vi "运维调试_CODCr.vi"() -> ()   [LabVIEW 2016, in "CODCr库.lvlib"]
uses:
  <vilib>/Utility/miscctls.llb/LVPointTypeDef.ctl
  <vilib>/ptbypt/NI_PtbyPt.lvlib
  <vilib>/Utility/config.llb/NI_LVConfig.lvlib
panel:
  out "数据时间":timestamp format="%<%Y/%m/%d %H:%M:%S>T"
  in  "质控参数":bool
  in  "仪器参数":bool
  in  "MB通信方式选择":enum16{"串口", "TCP"}(ring)
  in  "释放串口":bool
  in  "打开串口":bool
  in  "加标回收测试":bool
  in  "平行样测试":bool
  in  "定时启动":bool
  out "COM口":string
  in  "空白测试":bool
  in  "隐藏按钮":bool
  in  "写入消解温度时长":bool
  in  "保存KB值":bool
  in  "标样核查":bool
  out "启动时间":timestamp format="%<%Y/%m/%d %H:%M:%S>T"
  out "主循环次数":i32
  out "status":bool
  out "启动测量模式":T1(ring)
  out "曲线截距B":sgl format="%#_10g"
  out "曲线斜率K":sgl format="%#_10g"
  out "量程上限":sgl
  out "量程下限":sgl
  out "消解时长":u16
  out "消解温度":u16
  out "测量精度":u16
  out "测量结果":sgl
  out "标样参考值":sgl
  out "量程":u16
  out "工作状态":T1(ring)
  out "仪器时间":timestamp format="%<%X\n%x>T"
  out "关键参数区":T2
  out "状态告警区":T3 {"告警代码" items=["无告警", "缺试剂告警", "缺水样告警", "缺蒸馏水告警", "缺标液告警", "仪表漏液告警", "标定异常告警", "超量程告警", "加热异常", "低试剂预警", "超上限告警", "超下限告警", "仪表内部其他异常", "滴定异常告警", "电极异常告警", "量程切换告警", "参数设置告警", "PH电极电位异常", "电导率电极异常", "浊度光度异常", "溶解氧电极异常", "溶解氧光强异常", "温度异常告警", "PH异常告警", "溶解氧异常告警", "电导率异常告警", "浊度异常告警", "叶绿素异常告警", "藻密度异常告警", "蓝绿藻异常告警", "ORP异常告警", "氨氮异常告警", "清洁刷异常告警", "SD卡异常告警", "蓝牙异常告警", "Wifi异常告警", "流程异常告警"]; "故障代码" items=["无故障", "电机故障", "温度故障", "通讯故障", "滴定故障"]}
  out "测量数据区":T4 {"单位" items=["ug/L", "mg/L", "ppm", "mg/m3", "cm", "ppb", "ug/m3", "%", "nmol/mol", "umol/mol", "MPN/L", "MPN/100ml", "ng/m3", "NTU", "无量纲", "ms/cm", "us/cm", "℃", "mV", "万个/L"]}
  out "系统时间":timestamp format="%<%Y/%m/%d %H:%M:%S>T"
  in  "停止":bool
  in  "校时":bool
  in  "标样校准":bool
  in  "空白校准":bool
  in  "零点核查":bool
  in  "跨度核查":bool
  in  "水样测试":bool
  in  "返回":bool
  in  "设置":bool
  # "mg/L"
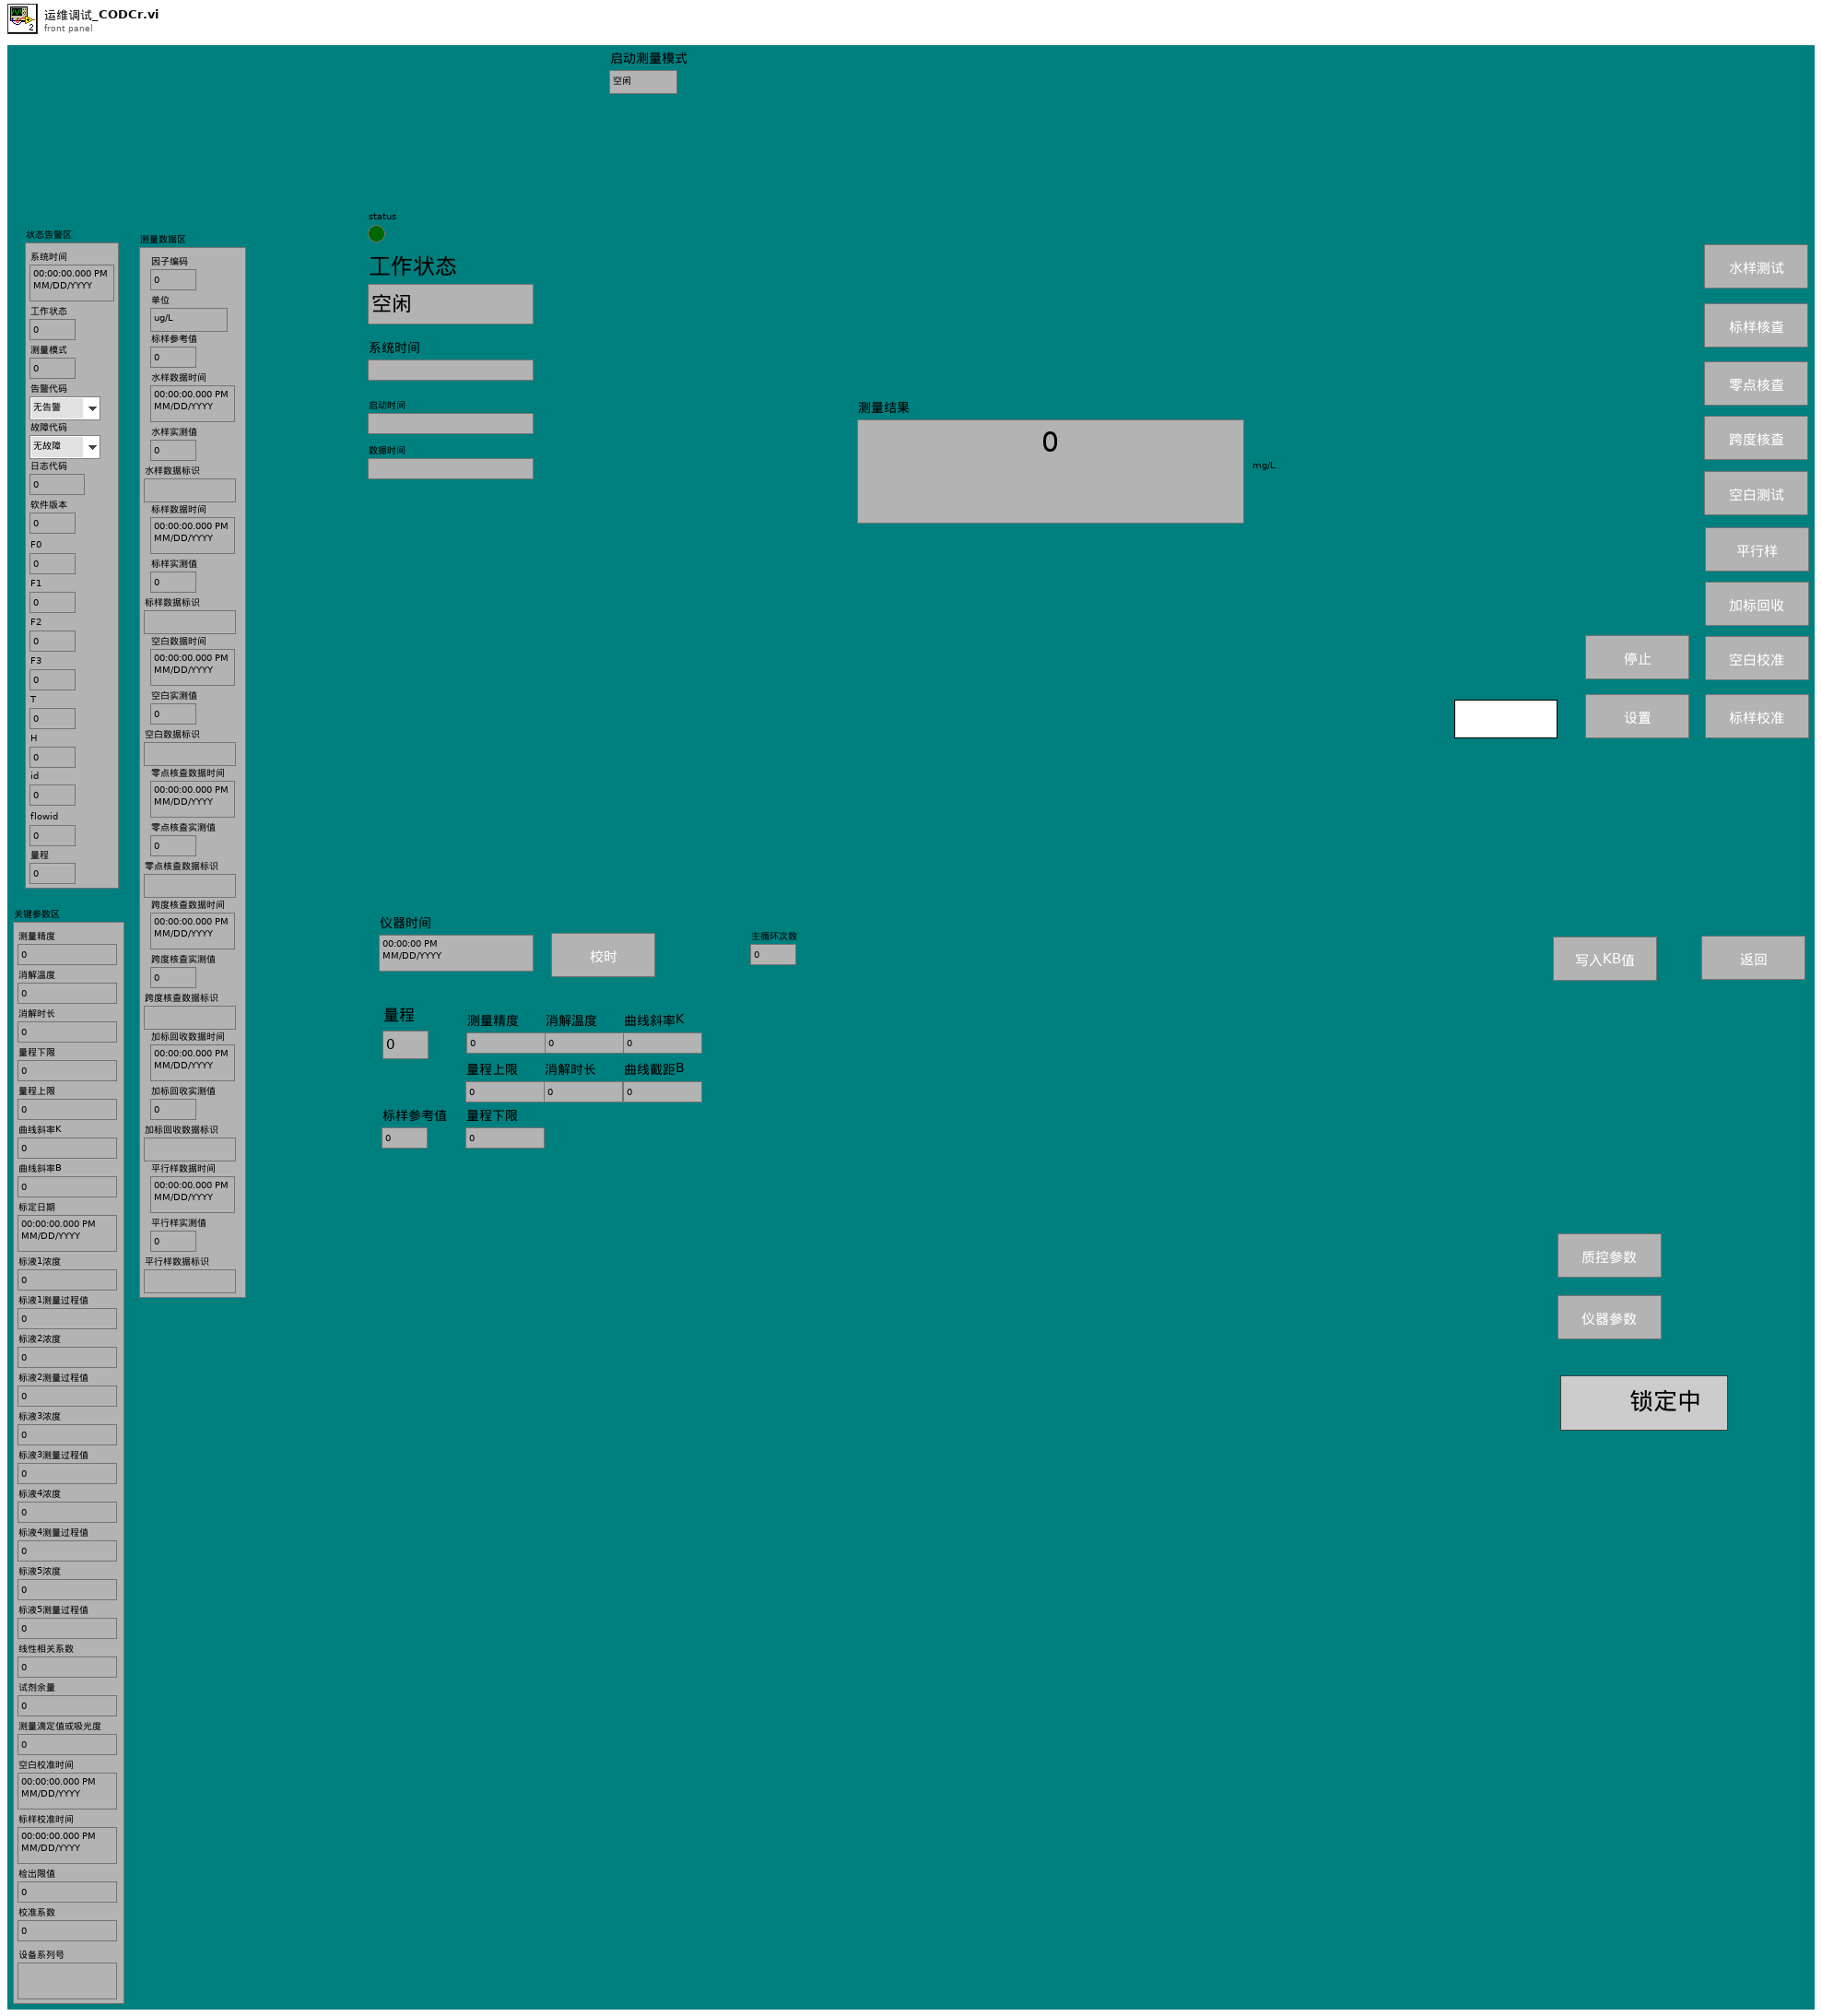
[diagram p1: front panel]
types:
  T1 = enum16{"空闲", "水样测试", "标样核查", "零点核查", "跨度核查", "空白测试", "平行样测试", "加标回收", "空白校准", "标样校准", "初始化（清洗）"}
  T2 = cluster{"测量精度":u16, "消解温度":u16, "消解时长":u16, "量程下限":sgl, "量程上限":sgl, "曲线斜率K":sgl, "曲线斜率B":sgl, "标定日期":timestamp, "标液1浓度":sgl, "标液1测量过程值":sgl, "标液2浓度":sgl, "标液2测量过程值":sgl, "标液3浓度":sgl, "标液3测量过程值":sgl, "标液4浓度":sgl, "标液4测量过程值":sgl, "标液5浓度":sgl, "标液5测量过程值":sgl, "线性相关系数":sgl, "试剂余量":u32, "测量滴定值或吸光度":sgl, "空白校准时间":timestamp, "标样校准时间":timestamp, "检出限值":sgl, "校准系数":sgl, "设备系列号":string}
  T3 = cluster{"系统时间":timestamp, "工作状态":u16, "测量模式":u16, "告警代码":u16, "故障代码":u16, "日志代码":u16, "软件版本":u16, "F0":sgl, "F1":sgl, "F2":sgl, "F3":sgl, "T":sgl, "H":sgl, "id":u16, "flowid":u16, "量程":u16}
  T4 = cluster{"因子编码":u32, "单位":u16, "标样参考值":sgl, "水样数据时间":timestamp, "水样实测值":sgl, "水样数据标识":string, "标样数据时间":timestamp, "标样实测值":sgl, "标样数据标识":string, "空白数据时间":timestamp, "空白实测值":sgl, "空白数据标识":string, "零点核查数据时间":timestamp, "零点核查实测值":sgl, "零点核查数据标识":string, "跨度核查数据时间":timestamp, "跨度核查实测值":sgl, "跨度核查数据标识":string, "加标回收数据时间":timestamp, "加标回收实测值":sgl, "加标回收数据标识":string, "平行样数据时间":timestamp, "平行样实测值":sgl, "平行样数据标识":string}
  T5 = cluster{"命令":string, "测量模式":enum16{"水样测量", "标样核查", "零点核查", "跨度核查", "空白测试", "加标回收", "平行样", "校零", "校标"}, "CODCr量程切换":enum32{"H", "L", "AUTO"}}
  T6 = typedef "LVPointTypeDef.ctl" = cluster{"Horizontal":i16, "Vertical":i16}
  T7 = typedef "NI_LVConfig.lvlib/Config Data RefNum.ctl" = refnum<k1>
  T8 = enum8{"Enabled", "Disabled", "Disabled and Grayed Out"}
  T9 = cluster{"运行模式":enum16{"维护模式", "常规模式", "应急模式", "质控模式"}}
  T10 = cluster{"时间标识":timestamp, "监测值":sgl, "单位":u16, "数据标识":string, "因子编码":u32, "标样参考值":sgl, "F0":sgl, "F1":sgl, "F2":sgl, "F3":sgl, "温度":sgl, "湿度":sgl, "量程标识":string, "LastTime":timestamp}
  T11 = cluster{"时间标识":timestamp, "设备":string, "日志信息":string}
  T12 = cluster{"时间标识":timestamp, "参数":string, "日志信息":string, "流程参数":string}
  T13 = cluster{"时间标识":timestamp, "设备":string, "日志信息":string, "流程参数":string}
  T14 = enum16{"水样测量", "标样核查", "零点核查", "跨度核查", "空白测试", "加标回收", "平行样", "校零", "校标"}
  T15 = cluster{"控制命令":enum16{"启动测量", "标样核查", "零点核查", "跨度核查", "空白测试", "平行样测试", "加标回收", "空白校准", "标样校准", "初始化（清洗）", "停止测试", "仪器重启", "校时", "模式设置", "测量间隔设置"}, "周期设置类型":enum16{"定点启动", "间隔启动"}, "定时功能启用":bool, "定时间隔":dbl, "24H周期设置":bool[], "零点核查时间":u16, "跨度核查时间":u16, "质控频次":enum16{"关闭", "每天", "星期一", "星期二", "星期三", "星期四", "星期五", "星期六", "星期日"}}
  T16 = cluster{"测量量程":dbl, "测量精度":dbl, "测量间隔":dbl, "消解温度":dbl, "消解时长":dbl, "空白校准时间":timestamp, "曲线截距":dbl, "曲线斜率":dbl, "测量检出限":dbl, "测量信号值":dbl, "线性相关系数":dbl, "二次多项式系数":dbl, "标样校准时间":timestamp, "稀释倍数":dbl, "三项式系数":dbl, "空白标定系数":dbl, "量程系数":dbl, "F0/ORPA":dbl, "F1/ORPB":dbl, "F2/ORPK":dbl, "F3":dbl, "F4":dbl, "F5":dbl, "F6":dbl, "F7":dbl, "X0/滴定数":dbl, "量程":dbl}
  T17 = cluster{"控制命令":enum16{"启动测量", "标样核查", "零点核查", "跨度核查", "空白测试", "平行样测试", "加标回收", "空白校准", "标样校准", "初始化（清洗）", "停止测试", "仪器重启", "校时", "模式设置", "测量间隔设置"}, "周期设置类型":enum16{"定点启动", "间隔启动"}, "定时功能启用":bool, "定时间隔":dbl, "24H周期设置":bool[], "空白核查时间":u16, "跨度核查时间":u16, "质控频次":enum16{"关闭", "每天", "星期一", "星期二", "星期三", "星期四", "星期五", "星期六", "星期日"}}
  T18 = cluster{"确定":bool, "测量量程":dbl, "测量精度":dbl, "测量间隔":dbl, "消解温度":dbl, "消解时长":dbl, "空白校准时间":timestamp, "曲线截距":dbl, "曲线斜率":dbl, "测量检出限":dbl, "测量信号值":dbl, "线性相关系数":dbl, "二次多项式系数":dbl, "标样校准时间":timestamp, "稀释倍数":dbl, "三项式系数":dbl, "空白标定系数":dbl, "量程系数":dbl, "F0/ORPA":dbl, "F1/ORPB":dbl, "F2/ORPK":dbl, "F3":dbl, "F4":dbl, "F5":dbl, "F6":dbl, "F7":dbl, "X0/滴定数":dbl, "量程":dbl}
  T19 = cluster{"跨度值":dbl, "零点标准液浓度":dbl, "跨度标准液浓度":dbl, "标准液标准浓度":dbl}
  T20 = cluster{"确定":bool, "跨度值":dbl, "零点标准液浓度":dbl, "跨度标准液浓度":dbl, "标准液标准浓度":dbl}
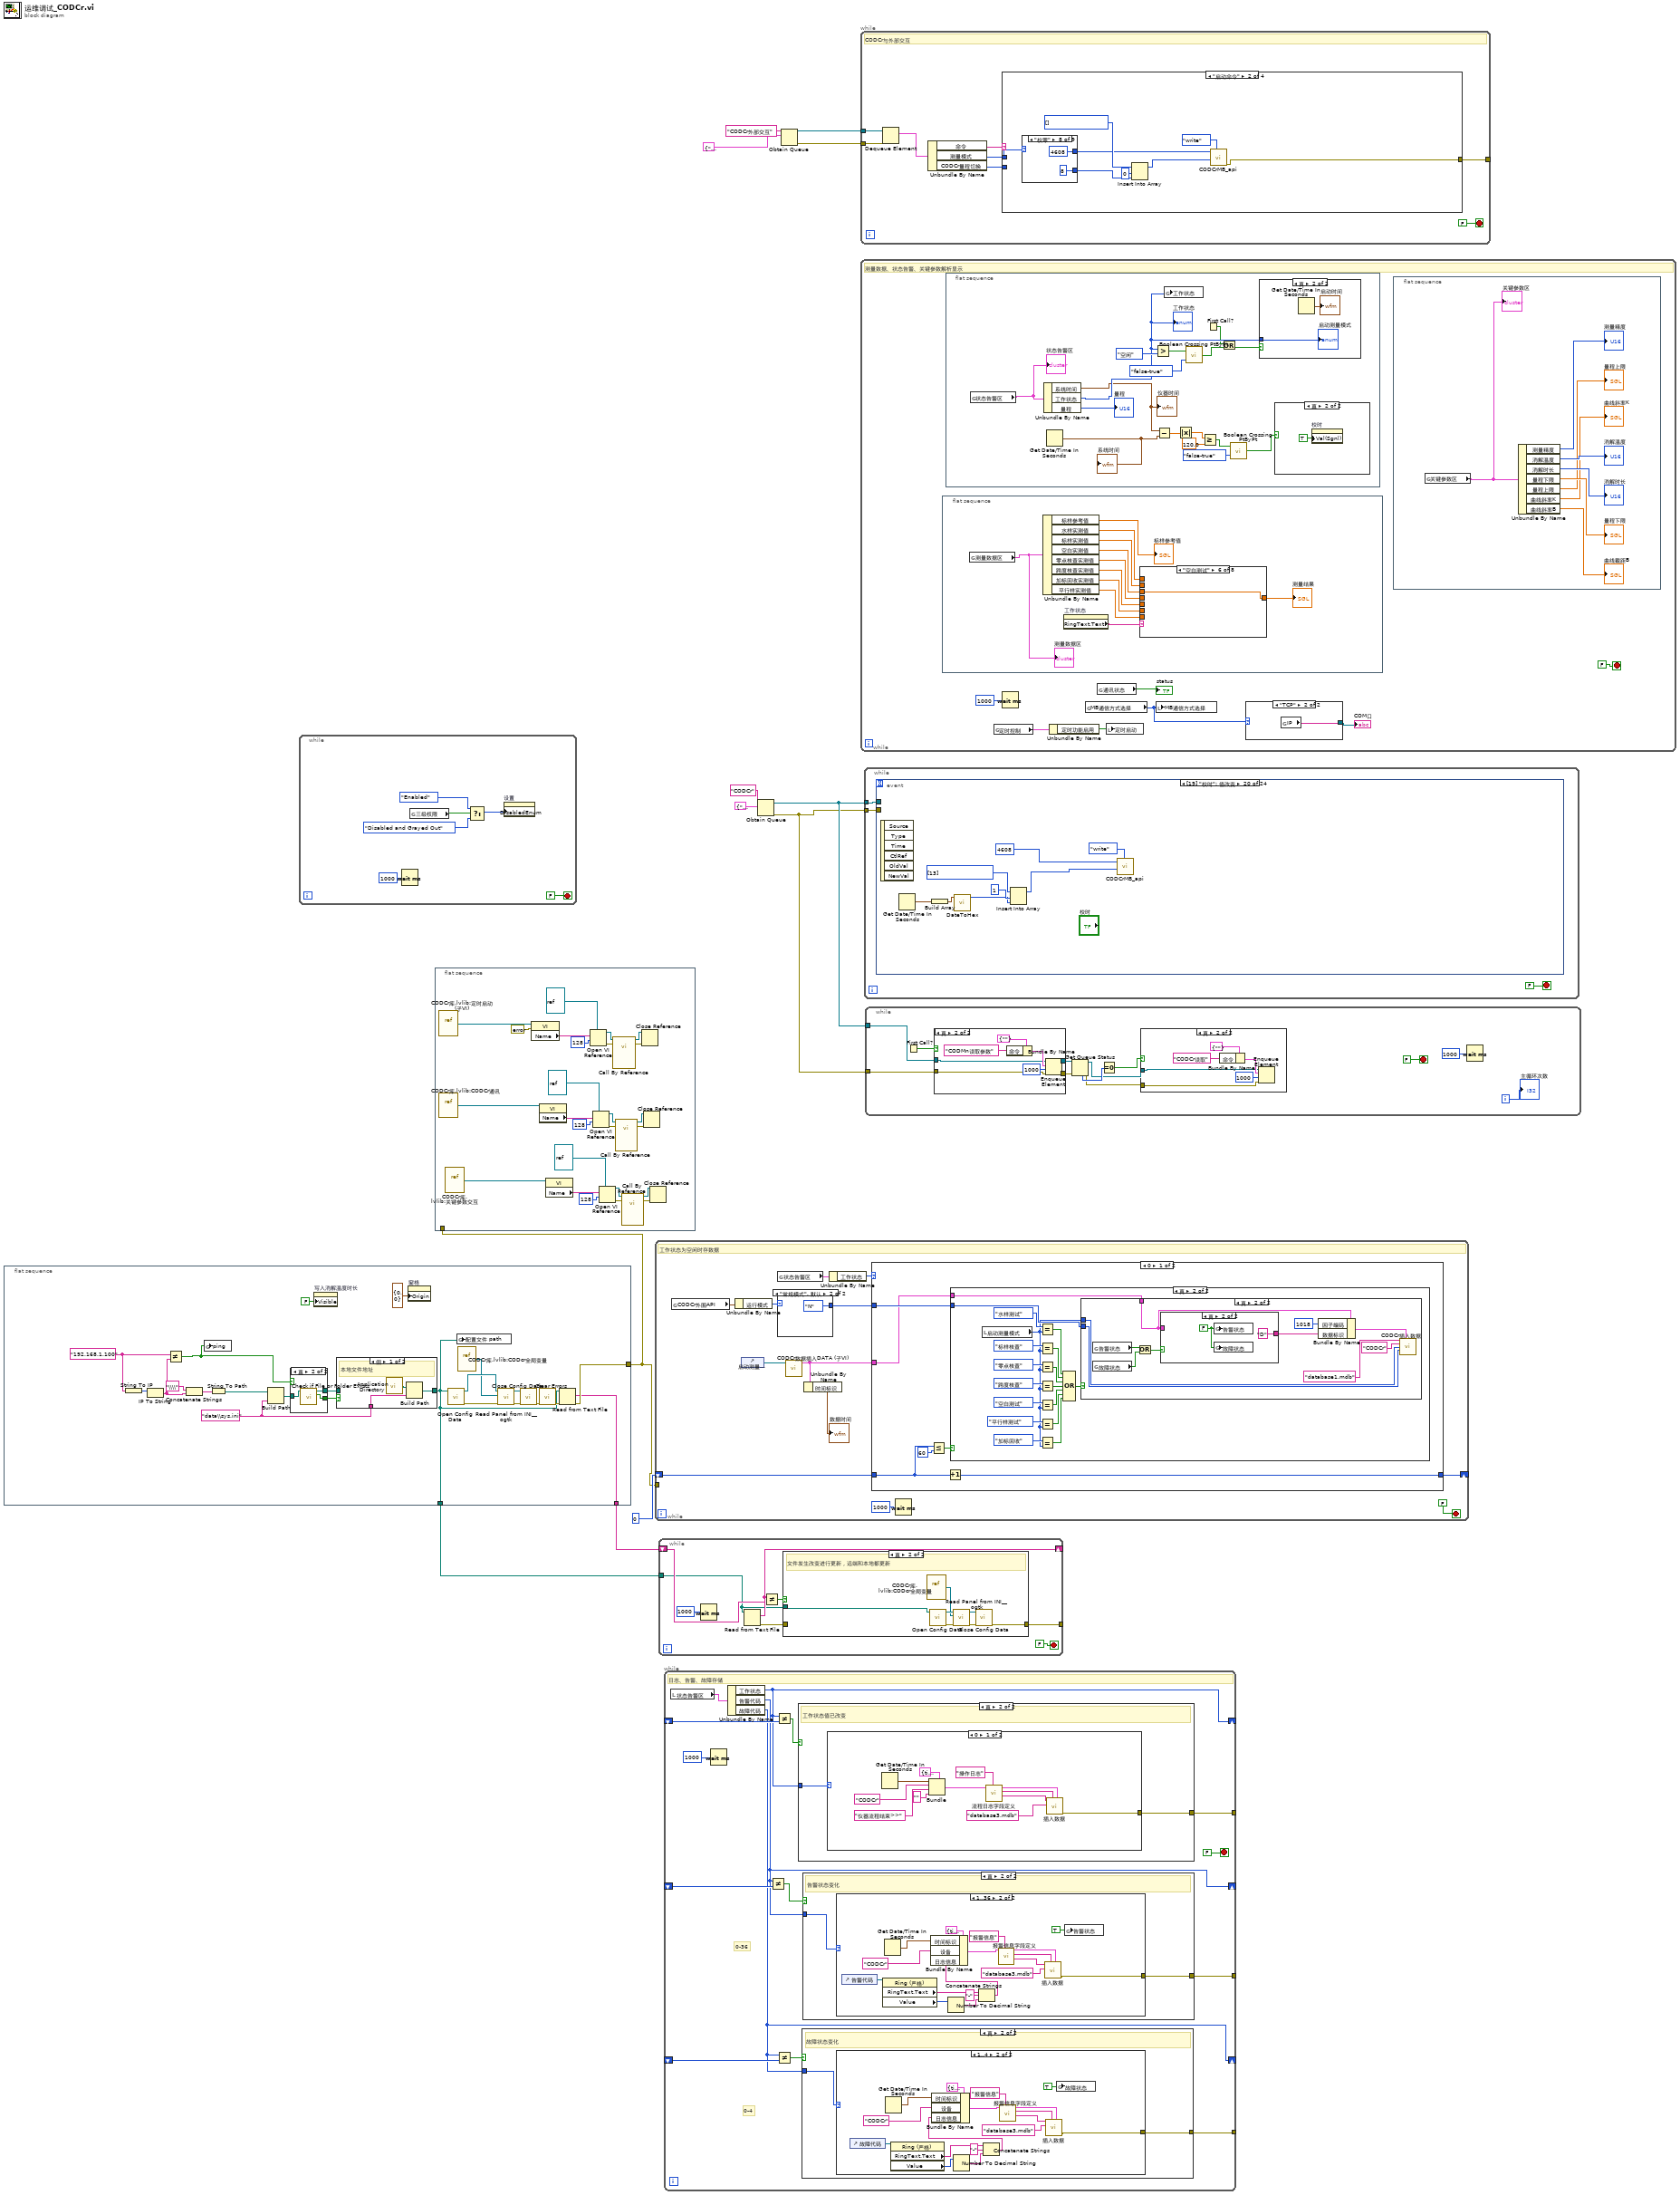
[diagram p0: block diagram]
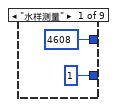
[diagram p6: hidden frame]
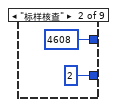
[diagram p7: hidden frame]
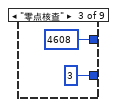
[diagram p8: hidden frame]
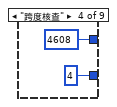
[diagram p9: hidden frame]
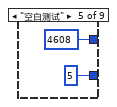
[diagram p10: hidden frame]
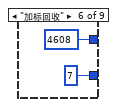
[diagram p11: hidden frame]
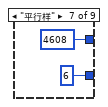
[diagram p12: hidden frame]
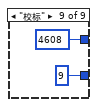
[diagram p13: hidden frame]
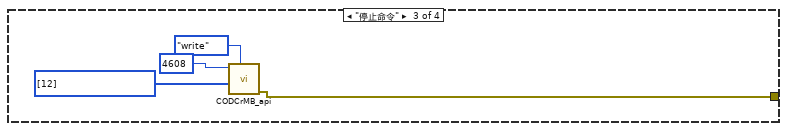
[diagram p14: hidden frame]
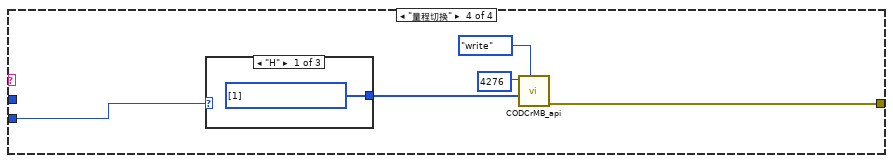
[diagram p15: hidden frame]
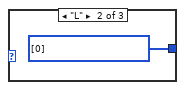
[diagram p16: hidden frame]
diagram:
  n1 = flat-sequence {
    tunnel: [w15] -> w1
    tunnel: [w14] -> w3
    tunnel: [w13] -> w2
    frame #0 {
      w33 = "data\\sys.ini" ("名称或相对路径")
      w18 = "192.168.1.100" ("名称")
      n2 = String To IP(1:w18) -> (0:w25:u32)
      n3 = IP To String(2:w25) -> (0:w22:string)  [unwired: 1 in]
      n4 = Not Equal?(x=w18, y=w22) -> (x != y?=w32:bool)
      n5 = Concatenate Strings("\\\\" ("字符串"), w22) -> (w23:string)
      n6 = global write "CODcr全局变量.vi" "ping"(w32) -> ()
      n7 = String To Path(string=w23) -> (path=w17:path)
      n8 = Build Path(base path=w17, name or relative path=w33) -> (appended path=w21:path)
      n9 = case shown="真" w32 {
        tunnel: w21 -> [w36 w40]
        tunnel: [w36 w39] -> w20
        tunnel: [FALSE w38] -> w19
        frame False {
        }
        frame True {
          n10 = call <vilib>:"Check if File or Folder Exists.vi"("path"=w40) -> ("file or folder exists?"=w38:bool, "dup path"=w39:path)  [unwired: 8 in, 1 out]
        }
      }
      n11 = property on="写入消解温度时长" class="Bool"("Visible"=FALSE ("可见")) -> ()  [unwired: 2 in, 2 out]
      n12 = case shown="假" w19 {
        tunnel: w20 -> [_ w44]
        tunnel: [w42 w44] -> w13
        tunnel: w33 -> [w41 _]
        frame False {
          # "本地文件地址"
          n13 = call <vilib>:"Application Directory.vi"() -> ("Application Directory"=w43:path)
          n14 = Build Path(base path=w43, name or relative path=w41) -> (appended path=w42:path)
        }
        frame True {
          # "网络共享地址"
        }
      }
      n15 = property on="窗格" class="Pane"("Origin"=T6 {"Horizontal"=0, "Vertical"=0} ("原点")) -> ()  [unwired: 2 in, 2 out]
      n16 = call <vilib>:"Open Config Data.vi"("configuration file path"=w13) -> ("error out"=w29:errorcluster, "refnum"=w28:T7)  [unwired: 8 in, 1 out]
      n17 = global write "CODcr全局变量.vi" "配置文件 path"(w13) -> ()
      n18 = vi-ref "CODCr库.lvlib:CODcr全局变量.vi"() -> (w16:refnum<vi>)
      n19 = call <userlib>:"Read Panel from INI__ogtk.vi"("error in (no error)"=w29, "VI ref"=w16, "refnum"=w28) -> ("error out"=w27:errorcluster, "refnum out"=w26:T7)  [unwired: 7 in]
      n20 = call <vilib>:"Close Config Data.vi"("error in (no error)"=w27, "refnum"=w26) -> ("error out"=w30:errorcluster)  [unwired: 8 in, 1 out]
      n21 = call <vilib>:"Clear Errors.vi"("error in (no error)"=w30) -> ("error out"=w31:errorcluster)  [unwired: 5 in, 1 out]
      n22 = Read from Text File(file (use dialog)=w13, error in=w31) -> (text=w14:string, error out=w15:errorcluster)  [unwired: 2 in, 2 out]
    }
  }
  n23 = while {
    stop <- FALSE stop-if-true
    n24 = Wait (ms)(milliseconds to wait=u32 1000 ("等待时间（毫秒）")) -> ()  [unwired: 1 out]
    n25 = global read "系统设置全局变量.vi" "三级权限"() -> (w48:bool)
    n26 = Select(t=T8."Enabled" ("禁用"), s=w48, f=T8."Disabled and Grayed Out" ("禁用")) -> (s? t:f=w45:T8)
    n27 = property on="设置" class="Bool"("DisabledEnum"=w45) -> ()  [unwired: 2 in, 2 out]
  }
  n28 = flat-sequence {
    tunnel: w1 -> [_]
    frame #0 {
      n29 = vi-ref "CODCr库.lvlib:定时启动 (子VI).vi"() -> (w59:refnum<vi>)
      n30 = vi-ref "CODCr库.lvlib:CODCr通讯.vi"() -> (w68:refnum<vi>)
      n31 = vi-ref "CODCr库.lvlib:关键参数交互.vi"() -> (w58:refnum<vi>)
      n32 = property class="VI"(reference=w59, error in=errorcluster {"status"=FALSE, "code"=0, "source"=""} ("错误输出")) -> ("Name"=w60:string)  [unwired: 2 out]
      n33 = property class="VI"(reference=w68) -> ("Name"=w69:string)  [unwired: 1 in, 2 out]
      n34 = property class="VI"(reference=w58) -> ("Name"=w57:string)  [unwired: 1 in, 2 out]
      n35 = Open VI Reference(type specifier VI Refnum (for type only)=refnum<vi> refnum, vi path=w60, options=128 ("选项")) -> (vi reference=w62:refnum<vi>, error out=w64:errorcluster)  [unwired: 3 in]
      n36 = Open VI Reference(type specifier VI Refnum (for type only)=refnum<vi> refnum, vi path=w69, options=128 ("选项")) -> (vi reference=w71:refnum<vi>, error out=w73:errorcluster)  [unwired: 3 in]
      n37 = Open VI Reference(type specifier VI Refnum (for type only)=refnum<vi> refnum, vi path=w57, options=128 ("选项")) -> (vi reference=w55:refnum<vi>, error out=w53:errorcluster)  [unwired: 3 in]
      n38 = call-by-ref "?"(reference=w62, error in=w64) -> (reference out=w66:refnum<vi>, error out=w65:errorcluster)  [unwired: 12 in]
      n39 = call-by-ref "?"(reference=w71, error in=w73) -> (reference out=w75:refnum<vi>, error out=w74:errorcluster)  [unwired: 12 in]
      n40 = call-by-ref "?"(reference=w55, error in=w53) -> (reference out=w51:refnum<vi>, error out=w52:errorcluster)  [unwired: 12 in]
      n41 = Close Reference(reference=w66, error in (no error)=w65) -> ()  [unwired: 1 out]
      n42 = Close Reference(reference=w75, error in (no error)=w74) -> ()  [unwired: 1 out]
      n43 = Close Reference(reference=w51, error in (no error)=w52) -> ()  [unwired: 1 out]
    }
  }
  n44 = while "While循环" {
    tunnel: w1 -> [_]
    shift-right: [w79] -> _
    shift-left: 0 -> [w80]
    stop <- FALSE stop-if-true
    # "工作状态为空闲时存数据"
    n45 = global read "CODCr外部API.vi" "CODCr外围API"() -> (w83:T9)
    n46 = Unbundle By Name(w83) -> ("运行模式"=w82:enum16{"维护模式", "常规模式", "应急模式", "质控模式"})
    n47 = control-ref of="启动测量模式"() -> (w78:refnum<vi>)
    n48 = global read "CODcr全局变量.vi" "状态告警区"() -> (w81:T3)
    n49 = case shown="\"常规模式\", 默认" w82 {
      tunnel: [enum16{"N", "M"}."M" ("数据类型") enum16{"N", "M"}."N" ("数据类型")] -> w84
      frame "维护模式" {
      }
      frame "常规模式", Default {
      }
    }
    n50 = call "CODCr数据插入DATA (子VI).vi"("Enum输入"=w78) -> ("data"=w77:T10)  [unwired: 10 in]
    n51 = Unbundle By Name(w77) -> ("时间标识"=→"数据时间":timestamp)
    n52 = Unbundle By Name(w81) -> ("工作状态"=w85:u16)
    n53 = case shown="0" w85 {
      tunnel: w84 -> [w95 _]
      tunnel: w80 -> [w93 _]
      tunnel: [w94 _] -> w79
      tunnel: w77 -> [w90 _]
      frame 0 {
        n54 = Less Or Equal?(x=w93, y=60) -> (x <= y?=w91:bool)
        n55 = Increment(x=w93) -> (x+1=w94:i32)
        n56 = case shown="真" w91 {
          tunnel: w95 -> [_ w113]
          tunnel: w90 -> [_ w96]
          frame False {
          }
          frame True {
            n57 = local read "启动测量模式"() -> (w105:T1)
            n58 = Equal?(x=T1."水样测试" ("启动测量模式"), y=w105) -> (x = y?=w104:bool)
            n59 = Equal?(x=T1."标样核查" ("启动测量模式"), y=w105) -> (x = y?=w103:bool)
            n60 = Equal?(x=T1."零点核查" ("启动测量模式"), y=w105) -> (x = y?=w102:bool)
            n61 = Equal?(x=T1."跨度核查" ("启动测量模式"), y=w105) -> (x = y?=w101:bool)
            n62 = Equal?(x=T1."空白测试" ("启动测量模式"), y=w105) -> (x = y?=w100:bool)
            n63 = Equal?(x=T1."平行样测试" ("启动测量模式"), y=w105) -> (x = y?=w99:bool)
            n64 = Equal?(x=T1."加标回收" ("启动测量模式"), y=w105) -> (x = y?=w98:bool)
            n65 = Compound Arithmetic op=OR(w104, w103, w102, w101, w100, w99, w98) -> (w97:bool)
            n66 = case shown="真" w97 {
              tunnel: w105 -> [_ w121]
              tunnel: w113 -> [_ w120]
              tunnel: w96 -> [_ w114]
              frame False {
              }
              frame True {
                n67 = global read "CODcr全局变量.vi" "告警状态"() -> (w118:bool)
                n68 = global read "CODcr全局变量.vi" "故障状态"() -> (w117:bool)
                n69 = Or(x=w118, y=w117) -> (x .or. y?=w116:bool)
                n70 = case shown="真" w116 {
                  tunnel: w114 -> [w126 _]
                  tunnel: [w125 "D" ("table")] -> w115
                  frame False {
                    n71 = Unbundle By Name(w126) -> ("数据标识"=w125:string)
                  }
                  frame True {
                    w127 = FALSE ("告警状态")
                    n72 = global write "CODcr全局变量.vi" "告警状态"(w127) -> ()
                    n73 = global write "CODcr全局变量.vi" "故障状态"(w127) -> ()
                  }
                }
                n74 = Bundle By Name(cluster=w114, "因子编码"=u32 1018, "数据标识"=w115) -> (w124:T10)
                n75 = call "CODCr插入数据.vi"("database"="database1.mdb", "data"=w124, "table"="CODCr", "测量模式"=w121, "数据类型"=w120) -> ()  [unwired: 10 in, 1 out]
              }
            }
          }
        }
      }
      frame 1, Default {
      }
    }
    n76 = Wait (ms)(milliseconds to wait=u32 1000 ("等待时间（毫秒）")) -> ()  [unwired: 1 out]
  }
  n77 = while {
    tunnel: [w135] -> _
    shift-right: [w133] -> _
    shift-left: w3 -> [w132]
    tunnel: w2 -> [w129]
    stop <- FALSE stop-if-true
    n78 = Wait (ms)(milliseconds to wait=u32 1000 ("等待时间（毫秒）")) -> ()  [unwired: 1 out]
    n79 = Read from Text File(file (use dialog)=w129) -> (text=w133:string, error out=w130:errorcluster)  [unwired: 3 in, 2 out]
    n80 = Not Equal?(x=w133, y=w132) -> (x != y?=w131:bool)
    n81 = case shown="真" w131 {
      tunnel: [w137 w144] -> w135
      tunnel: w129 -> [_ w138]
      tunnel: w130 -> [w137 _]
      frame False {
      }
      frame True {
        # "文件发生改变进行更新，远端和本地都更新"
        n82 = vi-ref "CODCr库.lvlib:CODcr全局变量.vi"() -> (w139:refnum<vi>)
        n83 = call <vilib>:"Open Config Data.vi"("configuration file path"=w138) -> ("error out"=w143:errorcluster, "refnum"=w142:T7)  [unwired: 8 in, 1 out]
        n84 = call <userlib>:"Read Panel from INI__ogtk.vi"("error in (no error)"=w143, "VI ref"=w139, "refnum"=w142) -> ("error out"=w141:errorcluster, "refnum out"=w140:T7)  [unwired: 7 in]
        n85 = call <vilib>:"Close Config Data.vi"("error in (no error)"=w141, "refnum"=w140) -> ("error out"=w144:errorcluster)  [unwired: 8 in, 1 out]
      }
    }
  }
  n86 = while {
    shift-right: [w155] -> _
    shift-left: _ -> [w157]
    tunnel: [w154] -> _
    shift-right: [w151] -> _
    shift-left: _ -> [w152]
    shift-right: [w147] -> _
    shift-left: _ -> [w149]
    tunnel: [w148] -> _
    tunnel: [w146] -> _
    stop <- FALSE stop-if-true
    # "0-4"
    # "0-36"
    # "日志、告警、故障存储"
    n87 = local read "状态告警区"() -> (w145:T3)
    n88 = Wait (ms)(milliseconds to wait=u32 1000 ("等待时间（毫秒）")) -> ()  [unwired: 1 out]
    n89 = Unbundle By Name(w145) -> ("工作状态"=w155:u16, "告警代码"=w151:u16, "故障代码"=w147:u16)
    n90 = Not Equal?(x=w151, y=w152) -> (x != y?=w153:bool)
    n91 = Not Equal?(x=w155, y=w157) -> (x != y?=w156:bool)
    n92 = Not Equal?(x=w147, y=w149) -> (x != y?=w150:bool)
    n93 = case shown="真" w156 {
      tunnel: w155 -> [_ w199]
      tunnel: [_ w198] -> w154
      frame False {
      }
      frame True {
        # "工作状态值已改变"
        n94 = case shown="0" w199 {
          tunnel: [w200 w215] -> w198
          frame 0 {
            n95 = Get Date/Time In Seconds() -> (seconds since 1Jan1904=w207:timestamp)
            n96 = Bundle(cluster=T12 {"时间标识"=timestamp(0 s since 1904-01-01), "参数"="", "日志信息"="", "流程参数"=""} ("data in"), "时间标识"=w207, "参数"="CODCr" ("table输入"), "日志信息"="仪器流程结束>>", "流程参数"="" ("table输入")) -> (w201:T12)
            n97 = call "流程日志字段定义.vi"("table输入"="操作日志", "data in"=w201) -> ("table输出"=w205:string, "columns"=w203:string[], "data out"=w202:T13)  [unwired: 7 in]
            n98 = call "插入数据.vi"("data"=w202, "columns"=w203, "database"="database3.mdb", "table"=w205) -> ("error out"=w200:errorcluster)  [unwired: 7 in]
          }
          frame 1, Default {
            n99 = property on="工作状态" class="Enum (严格)"() -> ("RingText.Text"=w212:string)  [unwired: 2 in, 2 out]
            n100 = Get Date/Time In Seconds() -> (seconds since 1Jan1904=w222:timestamp)
            n101 = Concatenate Strings("<<仪器流程开始" ("日志信息"), w212) -> (w213:string)
            n102 = Bundle(cluster=T12 {"时间标识"=timestamp(0 s since 1904-01-01), "参数"="", "日志信息"="", "流程参数"=""} ("data in"), "时间标识"=w222, "参数"="CODCr" ("table输入"), "日志信息"=w213, "流程参数"="" ("table输入")) -> (w221:T12)
            n103 = call "流程日志字段定义.vi"("table输入"="操作日志", "data in"=w221) -> ("table输出"=w219:string, "columns"=w217:string[], "data out"=w216:T13)  [unwired: 7 in]
            n104 = call "插入数据.vi"("data"=w216, "columns"=w217, "database"="database3.mdb", "table"=w219) -> ("error out"=w215:errorcluster)  [unwired: 7 in]
          }
        }
      }
    }
    n105 = case shown="真" w150 {
      tunnel: w147 -> [_ w161]
      tunnel: [_ w160] -> w146
      frame False {
      }
      frame True {
        # "故障状态变化"
        n106 = case shown="1..4" w161 {
          tunnel: [_ w168] -> w160
          frame 0, Default {
            # "无告警"
          }
          frame 1..4 {
            n107 = control-ref of="故障代码"() -> (w178:refnum<vi>)
            n108 = Get Date/Time In Seconds() -> (seconds since 1Jan1904=w176:timestamp)
            n109 = property class="Ring (严格)"(reference=w178) -> ("RingText.Text"=w165:string, "Value"=w166:u16)  [unwired: 1 in, 2 out]
            n110 = Number To Decimal String(number=w166) -> (decimal integer string=w163:string)  [unwired: 1 in]
            n111 = Concatenate Strings(w165, "-" ("字符串"), w163) -> (w164:string)
            n112 = Bundle By Name(cluster=T11 {"时间标识"=timestamp(0 s since 1904-01-01), "设备"="", "日志信息"=""} ("data in"), "时间标识"=w176, "设备"="CODCr" ("table输入"), "日志信息"=w164) -> (w175:T11)
            n113 = call "报警信息字段定义.vi"("table输入"="报警信息", "data in"=w175) -> ("table输出"=w170:string, "columns"=w169:string[], "data out"=w172:T11)  [unwired: 7 in]
            n114 = call "插入数据.vi"("data"=w172, "columns"=w169, "database"="database3.mdb", "table"=w170) -> ("error out"=w168:errorcluster)  [unwired: 7 in]
            n115 = global write "CODcr全局变量.vi" "故障状态"(TRUE ("告警状态")) -> ()
          }
        }
      }
    }
    n116 = case shown="真" w153 {
      tunnel: w151 -> [_ w180]
      tunnel: [_ w179] -> w148
      frame False {
      }
      frame True {
        # "告警状态变化"
        n117 = case shown="1..36" w180 {
          tunnel: [_ w190] -> w179
          frame 0, Default {
            # "无告警"
          }
          frame 1..36 {
            n118 = control-ref of="告警代码"() -> (w187:refnum<vi>)
            n119 = property class="Ring (严格)"(reference=w187) -> ("RingText.Text"=w185:string, "Value"=w184:u16)  [unwired: 1 in, 2 out]
            n120 = Get Date/Time In Seconds() -> (seconds since 1Jan1904=w189:timestamp)
            n121 = Number To Decimal String(number=w184) -> (decimal integer string=w181:string)  [unwired: 1 in]
            n122 = Concatenate Strings(w185, "-" ("字符串"), w181) -> (w183:string)
            n123 = Bundle By Name(cluster=T11 {"时间标识"=timestamp(0 s since 1904-01-01), "设备"="", "日志信息"=""} ("data in"), "时间标识"=w189, "设备"="CODCr" ("table输入"), "日志信息"=w183) -> (w191:T11)
            n124 = call "报警信息字段定义.vi"("table输入"="报警信息", "data in"=w191) -> ("table输出"=w196:string, "columns"=w197:string[], "data out"=w194:T11)  [unwired: 7 in]
            n125 = call "插入数据.vi"("data"=w194, "columns"=w197, "database"="database3.mdb", "table"=w196) -> ("error out"=w190:errorcluster)  [unwired: 7 in]
            n126 = global write "CODcr全局变量.vi" "告警状态"(TRUE ("告警状态")) -> ()
          }
        }
      }
    }
  }
  n127 = Obtain Queue(name (unnamed)="CODCr" ("名称（未命名）"), element data type=cluster{"命令":string} {"命令"="启用模块"} ("元素")) -> (queue out=w6:refnum<queue>, error out=w5:errorcluster)  [unwired: 3 in, 1 out]
  n128 = Obtain Queue(name (unnamed)="CODCr外部交互" ("名称（未命名）"), element data type=T5 {"命令"="启动命令", "测量模式"=enum."水样测量", "CODCr量程切换"=enum."AUTO"} ("元素")) -> (queue out=w8:refnum<queue>, error out=w7:errorcluster)  [unwired: 3 in, 1 out]
  n129 = while {
    tunnel: w8 -> [w231]
    tunnel: w7 -> [w230]
    tunnel: [w226] -> _
    stop <- FALSE stop-if-true
    # "CODCr与外部交互"
    n130 = Dequeue Element(queue=w231, error in (no error)=w230) -> (element=w232:T5)  [unwired: 1 in, 3 out]
    n131 = Unbundle By Name(w232) -> ("命令"=w229:string, "测量模式"=w228:T14, "CODCr量程切换"=w227:enum32{"H", "L", "AUTO"})
    n132 = case shown="\"启动命令\"" w229 {
      tunnel: w228 -> [_ w235 _ _]
      tunnel: w227 -> [_ _ _ w265]
      tunnel: [_ w234 w260 w264] -> w226
      frame "假", Default {
      }
      frame "启动命令" {
        n133 = case shown="\"校零\"" w235 {
          tunnel: [u16 4608 ("address") u16 4608 ("address") u16 4608 ("address") u16 4608 ("address") u16 4608 ("address") u16 4608 ("address") u16 4608 ("address") u16 4608 ("address") u16 4608 ("address")] -> w237
          tunnel: [u16 1 ("address") u16 2 ("address") u16 3 ("address") u16 4 ("address") u16 5 ("address") u16 7 ("address") u16 6 ("address") u16 8 ("address") u16 9 ("address")] -> w241
          frame "水样测量" {
          }
          frame "标样核查" {
          }
          frame "零点核查" {
          }
          frame "跨度核查" {
          }
          frame "空白测试" {
          }
          frame "加标回收" {
          }
          frame "平行样" {
          }
          frame "校零" {
          }
          frame "校标" {
          }
        }
        n134 = Insert Into Array(array=u16[] [] ("values"), index=0 ("索引"), new element=w241) -> (w236:u16[])
        n135 = call "CODCrMB_api.vi"("STEP"=enum16{"open", "read", "write", "close"}."write", "values"=w236, "starting address"=w237) -> ("error out"=w234:errorcluster)  [unwired: 6 in, 2 out]
      }
      frame "停止命令" {
        n136 = call "CODCrMB_api.vi"("STEP"=enum16{"open", "read", "write", "close"}."write", "values"=u16[] [12], "starting address"=u16 4608) -> ("error out"=w260:errorcluster)  [unwired: 6 in, 2 out]
      }
      frame "量程切换" {
        n137 = case shown="\"H\"" w265 {
          tunnel: [u16[] [1] ("values") u16[] [0] ("values") _] -> w268
          frame "H" {
          }
          frame "L" {
          }
          frame "AUTO", Default {
          }
        }
        n138 = call "CODCrMB_api.vi"("STEP"=enum16{"open", "read", "write", "close"}."write", "values"=w268, "starting address"=u16 4276) -> ("error out"=w264:errorcluster)  [unwired: 6 in, 2 out]
      }
    }
  }
  n139 = while {
    stop <- FALSE stop-if-true
    # "测量数据、状态告警、关键参数解析显示"
    n140 = flat-sequence {
      frame #0 {
        n141 = global read "CODcr全局变量.vi" "测量数据区"() -> (w308:T4)
        "测量数据区" <- w308
        n142 = Unbundle By Name(w308) -> ("标样参考值"=→"标样参考值":sgl, "水样实测值"=w316:sgl, "标样实测值"=w314:sgl, "空白实测值"=w311:sgl, "零点核查实测值"=w313:sgl, "跨度核查实测值"=w312:sgl, "加标回收实测值"=w309:sgl, "平行样实测值"=w310:sgl)
        n143 = property on="工作状态" class="Enum (严格)"() -> ("RingText.Text"=w317:string)  [unwired: 2 in, 2 out]
        n144 = case shown="\"空白测试\"" w317 {
          tunnel: w316 -> [_ w320 _ _ _ _ _ _]
          tunnel: [w319 w320 w321 w322 w323 w324 w325 w326] -> w315
          tunnel: w314 -> [_ _ w321 _ _ _ _ _]
          tunnel: w313 -> [_ _ _ w322 _ _ _ _]
          tunnel: w312 -> [_ _ _ _ w323 _ _ _]
          tunnel: w311 -> [_ _ _ _ _ w324 _ _]
          tunnel: w310 -> [_ _ _ _ _ _ w325 _]
          tunnel: w309 -> [_ _ _ _ _ _ _ w326]
          frame "空闲", Default {
            n145 = local read "测量结果"() -> (w319:sgl)
          }
          frame "水样测试" {
          }
          frame "标样核查" {
          }
          frame "零点核查" {
          }
          frame "跨度核查" {
          }
          frame "空白测试" {
          }
          frame "平行样测试" {
          }
          frame "加标回收" {
          }
        }
        "测量结果" <- w315
      }
    }
    n146 = flat-sequence {
      frame #0 {
        n147 = global read "CODcr全局变量.vi" "状态告警区"() -> (w296:T3)
        "状态告警区" <- w296
        n148 = Unbundle By Name(w296) -> ("系统时间"=w295:timestamp, "工作状态"=w299:u16, "量程"=→"量程":u16)
        "仪器时间" <- w295
        "工作状态" <- w299
        n149 = Get Date/Time In Seconds() -> (seconds since 1Jan1904=w294:timestamp)
        "系统时间" <- w294
        n150 = Greater?(x=w299, y=T1."空闲") -> (0:w303:bool)
        n151 = Subtract(x=w295, y=w294) -> (x-y=w293:dbl)
        n152 = global write "CODcr全局变量.vi" "工作状态"(w299) -> ()
        n153 = Absolute Value(x=w293) -> (abs(x)=w292:dbl)
        n154 = call <vilib>:"Boolean Crossing PtByPt.vi"("direction"=enum16{"either", "false-true", "true-false"}."false-true", "input"=w303) -> ("crossing"=w302:bool)  [unwired: 1 in]
        n155 = Greater Or Equal?(x=w292, y=120.0) -> (x >= y?=w290:bool)
        n156 = First Call?() -> (First Call?: T/F=w297:bool)
        n157 = Or(x=w297, y=w302) -> (x .or. y?=w298:bool)
        n158 = call <vilib>:"Boolean Crossing PtByPt.vi"("direction"=enum16{"either", "false-true", "true-false"}."false-true", "input"=w290) -> ("crossing"=w289:bool)  [unwired: 1 in]
        n159 = case shown="真" w298 {
          tunnel: w299 -> [_ w306]
          frame False {
          }
          frame True {
            n160 = Get Date/Time In Seconds() -> (seconds since 1Jan1904=→"启动时间":timestamp)
            "启动测量模式" <- w306
          }
        }
        n161 = case shown="真" w289 {
          frame False {
          }
          frame True {
            n162 = property on="校时" class="Bool (严格)"("Val(Sgnl)"=TRUE ("值(信号)")) -> ()  [unwired: 2 in, 2 out]
          }
        }
      }
    }
    n163 = global read "CODcr全局变量.vi" "定时控制"() -> (w272:T15)
    n164 = Wait (ms)(milliseconds to wait=u32 1000 ("等待时间（毫秒）")) -> ()  [unwired: 1 out]
    n165 = Unbundle By Name(w272) -> ("定时功能启用"=w271:bool)
    n166 = global read "CODcr全局变量.vi" "MB通信方式选择"() -> (w273:enum16{"串口", "TCP"})
    n167 = global read "CODcr全局变量.vi" "通讯状态"() -> (→"status":bool)
    n168 = local write "定时启动"(w271) -> ()
    n169 = local write "MB通信方式选择"(w273) -> ()
    n170 = case shown="\"TCP\"" w273 {
      tunnel: [w278 w279] -> w274
      frame "串口", Default {
        n171 = global read "CODcr全局变量.vi" "VISA Resource"() -> (w278:refnum<visa-resource-name>)
      }
      frame "TCP" {
        n172 = global read "CODcr全局变量.vi" "IP"() -> (w279:string)
      }
    }
    "COM口" <- w274
    n173 = flat-sequence {
      frame #0 {
        n174 = global read "CODcr全局变量.vi" "关键参数区"() -> (w280:T2)
        "关键参数区" <- w280
        n175 = Unbundle By Name(w280) -> ("测量精度"=→"测量精度":u16, "消解温度"=→"消解温度":u16, "消解时长"=→"消解时长":u16, "量程下限"=→"量程下限":sgl, "量程上限"=→"量程上限":sgl, "曲线斜率K"=→"曲线斜率K":sgl, "曲线斜率B"=→"曲线截距B":sgl)
      }
    }
  }
  n176 = while {
    tunnel: w6 -> [w328]
    tunnel: w5 -> [w327]
    stop <- FALSE stop-if-true
    n177 = event shown="[19] \"校时\": 值改变" {
      selector: _ -> [_ _ _ _ _ _ _ _ _ _ _ _ _ _ _ _ _ _ _ _ _ _ _ _]
      dyn-events: _ -> [_ _ _ _ _ _ _ _ _ _ _ _ _ _ _ _ _ _ _ _ _ _ _ _]
      timeout: _ -> [_ _ _ _ _ _ _ _ _ _ _ _ _ _ _ _ _ _ _ _ _ _ _ _]
      tunnel: w328 -> [_ _ _ _ _ _ _ _ _ _ _ _ _ _ _ w428 w447 _ _ _ w471 _ _ _]
      tunnel: w327 -> [_ _ _ _ _ _ _ _ _ _ _ _ _ _ _ w427 w446 _ _ _ w470 _ _ _]
      event Timeout {
        n178 = event-data() -> ()  [unwired: 1 in, 2 out]
      }
      event "水样测试": Value Change {
        n179 = event-data() -> ()  [unwired: 1 in, 6 out]
        n180 = local write "启动测量模式"(T1."水样测试" ("启动测量模式")) -> ()
        n181 = call "CODCrMB_api.vi"("STEP"=enum16{"open", "read", "write", "close"}."write", "values"=u16[] [1], "starting address"=u16 4608) -> ()  [unwired: 6 in, 3 out]
      }
      event "标样核查": Value Change {
        n182 = event-data() -> ()  [unwired: 1 in, 6 out]
        n183 = local write "启动测量模式"(T1."标样核查" ("启动测量模式")) -> ()
        n184 = call "CODCrMB_api.vi"("STEP"=enum16{"open", "read", "write", "close"}."write", "values"=u16[] [2], "starting address"=u16 4608) -> ()  [unwired: 6 in, 3 out]
      }
      event "零点核查": Value Change {
        n185 = event-data() -> ()  [unwired: 1 in, 6 out]
        n186 = local write "启动测量模式"(T1."零点核查" ("启动测量模式")) -> ()
        n187 = call "CODCrMB_api.vi"("STEP"=enum16{"open", "read", "write", "close"}."write", "values"=u16[] [3], "starting address"=u16 4608) -> ()  [unwired: 6 in, 3 out]
      }
      event "跨度核查": Value Change {
        n188 = event-data() -> ()  [unwired: 1 in, 6 out]
        n189 = local write "启动测量模式"(T1."跨度核查" ("启动测量模式")) -> ()
        n190 = call "CODCrMB_api.vi"("STEP"=enum16{"open", "read", "write", "close"}."write", "values"=u16[] [4], "starting address"=u16 4608) -> ()  [unwired: 6 in, 3 out]
      }
      event "空白测试": Value Change {
        n191 = event-data() -> ()  [unwired: 1 in, 6 out]
        n192 = local write "启动测量模式"(T1."空白测试" ("启动测量模式")) -> ()
        n193 = call "CODCrMB_api.vi"("STEP"=enum16{"open", "read", "write", "close"}."write", "values"=u16[] [5], "starting address"=u16 4608) -> ()  [unwired: 6 in, 3 out]
      }
      event "平行样测试": Value Change {
        n194 = event-data() -> ()  [unwired: 1 in, 6 out]
        n195 = local write "启动测量模式"(T1."平行样测试" ("启动测量模式")) -> ()
        n196 = call "CODCrMB_api.vi"("STEP"=enum16{"open", "read", "write", "close"}."write", "values"=u16[] [6], "starting address"=u16 4608) -> ()  [unwired: 6 in, 3 out]
      }
      event "加标回收测试": Value Change {
        n197 = event-data() -> ()  [unwired: 1 in, 6 out]
        n198 = local write "启动测量模式"(T1."加标回收" ("启动测量模式")) -> ()
        n199 = call "CODCrMB_api.vi"("STEP"=enum16{"open", "read", "write", "close"}."write", "values"=u16[] [7], "starting address"=u16 4608) -> ()  [unwired: 6 in, 3 out]
      }
      event "空白校准": Value Change {
        n200 = event-data() -> ()  [unwired: 1 in, 6 out]
        n201 = local write "启动测量模式"(T1."空白校准" ("启动测量模式")) -> ()
        n202 = call "CODCrMB_api.vi"("STEP"=enum16{"open", "read", "write", "close"}."write", "values"=u16[] [8], "starting address"=u16 4608) -> ()  [unwired: 6 in, 3 out]
      }
      event "标样校准": Value Change {
        n203 = event-data() -> ()  [unwired: 1 in, 6 out]
        n204 = local write "启动测量模式"(T1."标样校准" ("启动测量模式")) -> ()
        n205 = call "CODCrMB_api.vi"("STEP"=enum16{"open", "read", "write", "close"}."write", "values"=u16[] [9], "starting address"=u16 4608) -> ()  [unwired: 6 in, 3 out]
      }
      event "停止": Value Change {
        n206 = event-data() -> ()  [unwired: 1 in, 6 out]
        n207 = Two Button Dialog(message="确认是否停止？" ("消息"), 1:"否" ("F按钮名称（“取消”）"), 2:"是" ("T按钮名称（“确定”）")) -> (T button?=w366:bool)
        n208 = case shown="真" w366 {
          frame False {
          }
          frame True {
            n209 = Obtain Notifier(name (unnamed)="CODCr" ("名称（未命名）"), notification data type=FALSE) -> (notifier out=w374:refnum<notifier>, error out=w372:errorcluster)  [unwired: 2 in, 1 out]
            n210 = call "CODCrMB_api.vi"("STEP"=enum16{"open", "read", "write", "close"}."write", "values"=u16[] [12], "starting address"=u16 4608) -> ()  [unwired: 6 in, 3 out]
            n211 = Send Notification(notification=TRUE ("通知"), notifier=w374, error in (no error)=w372) -> (notifier out=w371:refnum<notifier>, error out=w370:errorcluster)
            n212 = Release Notifier(notifier=w371, error in (no error)=w370) -> ()  [unwired: 1 in, 3 out]
          }
        }
      }
      event "保存KB值": Value Change {
        n213 = event-data() -> ()  [unwired: 1 in, 6 out]
        n214 = local read "曲线截距B"() -> (w380:sgl)
        n215 = local read "曲线斜率K"() -> (w381:sgl)
        n216 = Build Array(w381, w380) -> (w386:sgl[])
        n217 = call "FloatToHex.vi"("浮点数"=w386) -> ("DCBA整形输出"=w383:u16[])  [unwired: 10 in]
        n218 = call "CODCrMB_api.vi"("STEP"=enum16{"open", "read", "write", "close"}."write", "values"=w383, "starting address"=u16 4263) -> ("error out"=w382:errorcluster)  [unwired: 6 in, 2 out]
        n219 = case shown="无错误" w382 {
          tunnel: w381 -> [w388 _]
          tunnel: w380 -> [w387 _]
          frame No Error {
            n220 = global read "CODcr全局变量.vi" "CODCr仪器参数"() -> (w390:T16)
            n221 = Bundle By Name(cluster=w390, "曲线截距"=w387, "曲线斜率"=w388) -> (w389:T16)
            n222 = global write "CODcr全局变量.vi" "CODCr仪器参数"(w389) -> ()
          }
          frame Error {
          }
        }
      }
      event "定时启动": Value Change {
        n223 = event-data() -> ()  [unwired: 1 in, 6 out]
        n224 = flat-sequence {
          frame #0 {
            n225 = global read "CODcr全局变量.vi" "定时控制"() -> (w392:T15)
            n226 = call "周期设置.vi"("定时控制输入"=w392) -> ("定时控制输出"=w391:T17)  [unwired: 10 in]
            n227 = global write "CODcr全局变量.vi" "定时控制"(w391) -> ()
          }
          frame #1 {
            n228 = call "配置文件保存.vi"() -> ()  [unwired: 12 in]
          }
        }
      }
      event "仪器参数": Value Change {
        n229 = event-data() -> ()  [unwired: 1 in, 6 out]
        n230 = global read "CODcr全局变量.vi" "CODCr仪器参数"() -> (w394:T16)
        n231 = call "仪器参数设置.vi"("氨氮仪器参数"=w394) -> ("仪器参数设置输出"=w393:T18)  [unwired: 10 in]
        n232 = Unbundle By Name(w393) -> ("确定"=w395:bool)
        n233 = case shown="真" w395 {
          tunnel: w394 -> [_ w397]
          tunnel: w393 -> [_ w396]
          frame False {
          }
          frame True {
            n234 = flat-sequence {
              tunnel: w397 -> [w414]
              tunnel: w396 -> [w413]
              frame #0 {
                n235 = Unbundle By Name(w413) -> ("测量量程"=w412:dbl, "测量精度"=w411:dbl, "测量间隔"=w410:dbl, "消解温度"=w409:dbl, "消解时长"=w408:dbl, "空白校准时间"=w407:timestamp, "曲线截距"=w406:dbl, "曲线斜率"=w405:dbl, "测量检出限"=w404:dbl, "测量信号值"=w403:dbl, "线性相关系数"=w402:dbl, "二次多项式系数"=w401:dbl, "标样校准时间"=w400:timestamp, "稀释倍数"=w399:dbl)
                n236 = Bundle By Name(cluster=w414, "测量量程"=w412, "测量精度"=w411, "测量间隔"=w410, "消解温度"=w409, "消解时长"=w408, "空白校准时间"=w407, "曲线截距"=w406, "曲线斜率"=w405, "测量检出限"=w404, "测量信号值"=w403, "线性相关系数"=w402, "二次多项式系数"=w401, "标样校准时间"=w400, "稀释倍数"=w399) -> (w398:T16)
                n237 = global write "CODcr全局变量.vi" "CODCr仪器参数"(w398) -> ()
              }
              frame #1 {
                n238 = call "配置文件保存.vi"() -> ()  [unwired: 12 in]
              }
            }
          }
        }
      }
      event "质控参数": Value Change {
        n239 = event-data() -> ()  [unwired: 1 in, 6 out]
        n240 = global read "CODcr全局变量.vi" "质控参数设置"() -> (w416:T19)
        n241 = call "质控参数设置.vi"("质控参数设置"=w416) -> ("输出簇"=w415:T20)  [unwired: 10 in]
        n242 = Unbundle By Name(w415) -> ("确定"=w417:bool)
        n243 = case shown="真" w417 {
          tunnel: w416 -> [_ w419]
          tunnel: w415 -> [_ w418]
          frame False {
          }
          frame True {
            n244 = flat-sequence {
              tunnel: w419 -> [w426]
              tunnel: w418 -> [w425]
              frame #0 {
                n245 = Unbundle By Name(w425) -> ("跨度值"=w423:dbl, "零点标准液浓度"=w422:dbl, "跨度标准液浓度"=w421:dbl, "标准液标准浓度"=w420:dbl)
                n246 = Bundle By Name(cluster=w426, "跨度值"=w423, "零点标准液浓度"=w422, "跨度标准液浓度"=w421, "标准液标准浓度"=w420) -> (w424:T19)
                n247 = global write "CODcr全局变量.vi" "质控参数设置"(w424) -> ()
              }
              frame #1 {
                n248 = call "配置文件保存.vi"() -> ()  [unwired: 12 in]
              }
            }
          }
        }
      }
      event "打开串口": Value Change {
        n249 = event-data() -> ()  [unwired: 1 in, 6 out]
        n250 = flat-sequence {
          tunnel: w428 -> [w430]
          tunnel: w427 -> [w429]
          frame #0 {
            n251 = global read "CODcr全局变量.vi" "VISA Resource"() -> (w437:refnum<visa-resource-name>)
            n252 = global read "CODcr全局变量.vi" "PORT"() -> (w431:string)
            n253 = global read "CODcr全局变量.vi" "IP"() -> (w432:string)
            n254 = call "串口配置.vi"("PORT"=w431, "IP"=w432, "请选择串口:"=w437) -> ("PORT 2"=w433:string, "IP 2"=w434:string, "确认 2"=w436:bool, "VISA资源名称 2"=w435:refnum<visa-resource-name>)  [unwired: 5 in]
            n255 = case shown="真" w436 {
              tunnel: w435 -> [_ w440]
              tunnel: w430 -> [_ w442]
              tunnel: w429 -> [_ w441]
              tunnel: w434 -> [_ w439]
              tunnel: w433 -> [_ w438]
              frame False {
              }
              frame True {
                n256 = global write "CODcr全局变量.vi" "VISA Resource"(w440) -> ()
                n257 = global write "CODcr全局变量.vi" "PORT"(w438) -> ()
                n258 = global write "CODcr全局变量.vi" "IP"(w439) -> ()
                n259 = Bundle By Name(cluster=cluster{"命令":string} {"命令"=""} ("元素"), "命令"="启用模块" ("名称（未命名）")) -> (w443:cluster{"命令":string})
                n260 = Enqueue Element(queue=w442, element=w443, error in (no error)=w441) -> ()  [unwired: 1 in, 3 out]
              }
            }
          }
          frame #1 {
            n261 = call "配置文件保存.vi"() -> ()  [unwired: 12 in]
          }
        }
      }
      event "释放串口": Value Change {
        n262 = event-data() -> ()  [unwired: 1 in, 6 out]
        n263 = Two Button Dialog(message="确认是否释放串口，释放串口将导致通信失败！" ("消息")) -> (T button?=w448:bool)  [unwired: 2 in]
        n264 = case shown="真" w448 {
          tunnel: w447 -> [_ w451]
          tunnel: w446 -> [_ w450]
          frame False {
          }
          frame True {
            n265 = Bundle By Name(cluster=cluster{"命令":string} {"命令"=""} ("元素"), "命令"="停用模块" ("名称（未命名）")) -> (w452:cluster{"命令":string})
            n266 = Enqueue Element(queue=w451, element=w452, error in (no error)=w450) -> ()  [unwired: 1 in, 3 out]
          }
        }
      }
      event "MB通信方式选择": Value Change {
        n267 = event-data() -> ()  [unwired: 1 in, 6 out]
        n268 = flat-sequence {
          frame #0 {
            n269 = global write "CODcr全局变量.vi" "MB通信方式选择"("MB通信方式选择") -> ()
          }
          frame #1 {
            n270 = call "配置文件保存.vi"() -> ()  [unwired: 12 in]
          }
        }
      }
      event "写入消解温度时长": Value Change {
        n271 = event-data() -> ()  [unwired: 1 in, 6 out]
        n272 = local read "消解时长"() -> (w460:u16)
        n273 = local read "消解温度"() -> (w461:u16)
        n274 = Build Array(w461, w460) -> (w459:u16[])
        n275 = call "WordToHex.vi"("WORD"=w459) -> ("数组"=w456:u16[])  [unwired: 10 in]
        n276 = call "CODCrMB_api.vi"("STEP"=enum16{"open", "read", "write", "close"}."write", "values"=w456, "starting address"=u16 4257) -> ()  [unwired: 6 in, 3 out]
      }
      event "校时": Value Change {
        n277 = event-data() -> ()  [unwired: 1 in, 6 out]
        n278 = Get Date/Time In Seconds() -> (seconds since 1Jan1904=w469:timestamp)
        n279 = Build Array(w469) -> (w466:timestamp[])
        n280 = call "DateToHex.vi"("DATE"=w466) -> ("数组"=w465:u16[])  [unwired: 10 in]
        n281 = Insert Into Array(array=u16[] [13] ("values"), index=1 ("索引"), new element=w465) -> (w462:u16[])
        n282 = call "CODCrMB_api.vi"("STEP"=enum16{"open", "read", "write", "close"}."write", "values"=w462, "starting address"=u16 4608) -> ()  [unwired: 6 in, 3 out]
      }
      event "设置": Value Change {
        n283 = event-data() -> ()  [unwired: 1 in, 6 out]
        n284 = property on="窗格" class="Pane"("Origin"=T6 {"Horizontal"=0, "Vertical"=728} ("原点")) -> ()  [unwired: 2 in, 2 out]
        n285 = Bundle By Name(cluster=cluster{"命令":string} {"命令"=""} ("元素"), "命令"="CODCr读取参数" ("名称（未命名）")) -> (w472:cluster{"命令":string})
        n286 = Enqueue Element(queue=w471, element=w472, error in (no error)=w470) -> ()  [unwired: 1 in, 3 out]
      }
      event "返回": Value Change {
        w476 = FALSE ("可见")
        n287 = event-data() -> ()  [unwired: 1 in, 6 out]
        n288 = property on="窗格" class="Pane"("Origin"=T6 {"Horizontal"=0, "Vertical"=0} ("原点")) -> ()  [unwired: 2 in, 2 out]
        n289 = property on="写入消解温度时长" class="Bool"("Visible"=w476) -> ()  [unwired: 2 in, 2 out]
        n290 = property on="释放串口" class="Bool"("Visible"=w476) -> ()  [unwired: 2 in, 2 out]
        n291 = property on="打开串口" class="Bool"("Visible"=w476) -> ()  [unwired: 2 in, 2 out]
        n292 = property on="MB通信方式选择" class="Enum (严格)"("Visible"=w476) -> ()  [unwired: 2 in, 2 out]
      }
      event "曲线斜率K", "曲线截距B", "消解温度", "消解时长": Mouse Down {
        n293 = event-data() -> ("CtlRef"=w480:refnum<vi>)  [unwired: 1 in, 7 out]
        n294 = property class="DigNum"(reference=w480) -> (reference out=w481:refnum<vi>, "Value"=w479:variant)  [unwired: 1 in, 1 out]
        n295 = Variant To Data(Variant=w479) -> (data=w478:sgl)  [unwired: 2 in, 1 out]
        n296 = call "CODCR数字键盘.vi"("OldNumber"=w478) -> ("NewNumber"=w482:sgl)
        n297 = property class="DigNum"(reference=w481, "Value"=w482) -> ()  [unwired: 1 in, 2 out]
      }
      event "隐藏按钮": Value Change {
        n298 = event-data() -> ("NewVal"=w483:bool)  [unwired: 1 in, 5 out]
        n299 = property on="写入消解温度时长" class="Bool"("Visible"=w483) -> ()  [unwired: 2 in, 2 out]
        n300 = property on="释放串口" class="Bool"("Visible"=w483) -> ()  [unwired: 2 in, 2 out]
        n301 = property on="打开串口" class="Bool"("Visible"=w483) -> ()  [unwired: 2 in, 2 out]
        n302 = property on="MB通信方式选择" class="Enum (严格)"("Visible"=w483) -> ()  [unwired: 2 in, 2 out]
      }
    }
  }
  n303 = while {
    tunnel: w6 -> [w485]
    tunnel: w5 -> [w484]
    i -> [w493]
    stop <- FALSE stop-if-true
    n304 = First Call?() -> (First Call?: T/F=w488:bool)
    n305 = case shown="真" w488 {
      tunnel: w485 -> [w497 w502]
      tunnel: w484 -> [w496 w501]
      tunnel: [w497 w500] -> w487
      tunnel: [w496 w499] -> w486
      frame False {
      }
      frame True {
        n306 = Bundle By Name(cluster=cluster{"命令":string} {"命令"=""} ("元素"), "命令"="CODMn读取参数" ("名称（未命名）")) -> (w505:cluster{"命令":string})
        n307 = Enqueue Element(queue=w502, element=w505, timeout in ms (-1)=1000 ("超时毫秒(-1)"), error in (no error)=w501) -> (queue out=w500:refnum<queue>, error out=w499:errorcluster)  [unwired: 1 out]
      }
    }
    n308 = Get Queue Status(queue=w487, error in (no error)=w486) -> (queue out=w491:refnum<queue>, error out=w490:errorcluster, # elements in queue=w492:i32)  [unwired: 1 in, 5 out]
    n309 = Equal To 0?(x=w492) -> (x = 0?=w489:bool)
    n310 = case shown="真" w489 {
      tunnel: w491 -> [_ w507]
      tunnel: w490 -> [_ w506]
      frame False {
      }
      frame True {
        n311 = Bundle By Name(cluster=cluster{"命令":string} {"命令"=""} ("元素"), "命令"="CODCr读取" ("名称（未命名）")) -> (w509:cluster{"命令":string})
        n312 = Enqueue Element(queue=w507, element=w509, timeout in ms (-1)=1000 ("超时毫秒(-1)"), error in (no error)=w506) -> ()  [unwired: 3 out]
      }
    }
    n313 = Wait (ms)(milliseconds to wait=u32 1000 ("等待时间（毫秒）")) -> ()  [unwired: 1 out]
    "主循环次数" <- w493
  }
